vi "ui_Library Two Button Dialog.vi"(1 "F button name (\"Cancel\")":string="Cancel", 2 "T button name (\"OK\")":string="OK", 3 "message":string) -> (0 "T button?":bool)   [LabVIEW 2012]
doc: "Drop-in replacement for LabVIEW's \"Two Button Dialog\" which, at least up to LabVIEW version 7.1, has the nasty property that it blocks the user interface thread while open. The UI thread is required not just for display updates but also for VI loading and instantiation. Thus, using the standard \"Two Button Dialog\" might prevent essential background tasks from doing their job. Since this subVI is implemented in LabVIEW, it does not suffer from this problem. Its connector pane layout is identical so that a simple diagram replace will work."
panel:
  out "message box":string
  in  "F button":bool
  in  "T button":bool
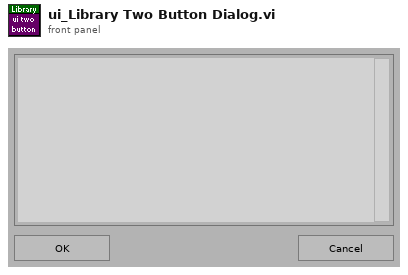
[diagram p1: front panel]
types:
  T1 = typedef "eventvkey.ctl" = enum16{"ASCII", "Enter", "Return", "Shift", "Ctrl", "Alt", "Cmd", "Opt", "Caps", "NumLock", "Clear", "Break", "Up", "Down", "Left", "Right", "Insert", "Delete", "Home", "End", "PageUp", "PageDown", "Escape", "Help", "Pause", "ScrollLock", "F1", "F2", "F3", "F4", "F5", "F6", "F7", "F8", "F9", "F10", "F11", "F12", "F13", "F14", "F15", "F16", "F17", "F18", "F19", "F20", "F21", "F22", "F23", "F24", "Play", "VolumeUp", "VolumeDown", "Mute", "Two Byte Char"}
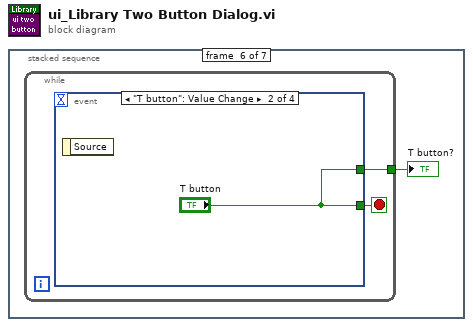
[diagram p0: block diagram]
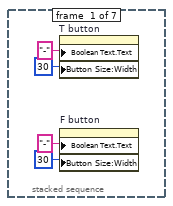
[diagram p2: hidden frame]
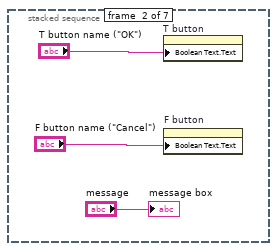
[diagram p3: hidden frame]
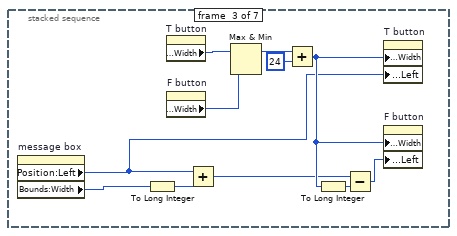
[diagram p4: hidden frame]
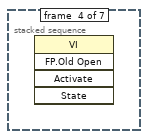
[diagram p5: hidden frame]
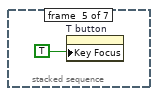
[diagram p6: hidden frame]
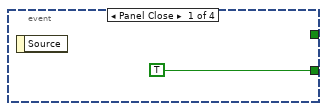
[diagram p7: hidden frame]
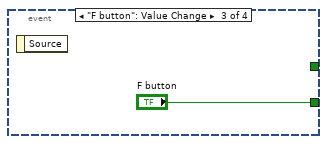
[diagram p8: hidden frame]
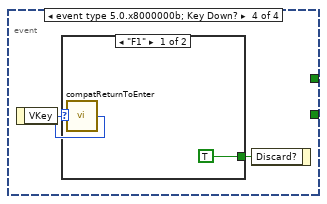
[diagram p9: hidden frame]
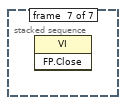
[diagram p11: hidden frame]
diagram:
  n1 = stacked-sequence {
    frame #0 {
      n2 = property on="T button" class="Bool"("Boolean Text.Text"="-", "Button Size:Width"=u32 30) -> ()  [unwired: 2 in, 2 out]
      n3 = property on="F button" class="Bool"("Boolean Text.Text"="-", "Button Size:Width"=u32 30) -> ()  [unwired: 2 in, 2 out]
    }
    frame #1 {
      n4 = property on="T button" class="Bool"("Boolean Text.Text"="T button name (\"OK\")") -> ()  [unwired: 2 in, 2 out]
      n5 = property on="F button" class="Bool"("Boolean Text.Text"="F button name (\"Cancel\")") -> ()  [unwired: 2 in, 2 out]
      "message box" <- "message"
    }
    frame #2 {
      n6 = property on="message box" class="Str"() -> ("Position:Left"=w9:i32, "Bounds:Width"=w8:u32)  [unwired: 2 in, 2 out]
      n7 = To Long Integer(number=w8) -> (32bit integer=w14:i32)
      n8 = property on="T button" class="Bool"() -> ("Button Size:Width"=w18:u32)  [unwired: 2 in, 2 out]
      n9 = property on="F button" class="Bool"() -> ("Button Size:Width"=w17:u32)  [unwired: 2 in, 2 out]
      n10 = Add(x=w9, y=w14) -> (x+y=w12:i32)
      n11 = Max & Min(x=w18, y=w17) -> (max(x,y)=w16:u32)  [unwired: 1 out]
      n12 = Add(x=w16, y=u32 24) -> (x+y=w13:u32)
      n13 = To Long Integer(number=w13) -> (32bit integer=w11:i32)
      n14 = Subtract(x=w12, y=w11) -> (x-y=w10:i32)
      n15 = property on="T button" class="Bool"("Button Size:Width"=w13, "Position:Left"=w9) -> ()  [unwired: 2 in, 2 out]
      n16 = property on="F button" class="Bool"("Button Size:Width"=w13, "Position:Left"=w10) -> ()  [unwired: 2 in, 2 out]
    }
    frame #3 {
      n17 = invoke class="VI" method="FP.Old Open"() -> ()  [unwired: 5 in, 5 out]
    }
    frame #4 {
      n18 = property on="T button" class="Bool"("Key Focus"=TRUE) -> ()  [unwired: 2 in, 2 out]
    }
    frame #5 {
      n19 = while {
        tunnel: [w22] -> w20
        stop <- w21 stop-if-true
        n20 = event shown="[1] \"T button\": Value Change" {
          selector: _ -> [_ _ _ _]
          dyn-events: _ -> [_ _ _ _]
          timeout: _ -> [_ _ _ _]
          tunnel: [_ "T button" _ _] -> w22
          tunnel: [TRUE "T button" "F button" _] -> w21
          event Panel Close {
            n21 = event-data() -> ()  [unwired: 1 in, 1 out]
          }
          event "T button": Value Change {
            n22 = event-data() -> ()  [unwired: 1 in, 1 out]
          }
          event "F button": Value Change {
            n23 = event-data() -> ()  [unwired: 1 in, 1 out]
          }
          event event type 5.0.x8000000b; Key Down? {
            n24 = event-data() -> ("VKey"=w26:T1)  [unwired: 1 in]
            n25 = call <vilib>:"compatReturnToEnter.vi"("VKey"=w26) -> ("VKey"=w28:T1)
            n26 = case shown="\"F1\"" w28 {
              tunnel: [TRUE ("Discard?") _] -> w27
              frame "F1" {
              }
              frame Default {
              }
            }
            n27 = event-data("Discard?"=w27) -> ()  [unwired: 1 in, 1 out]
          }
        }
      }
      "T button?" <- w20
    }
    frame #6 {
      n28 = invoke class="VI" method="FP.Close"() -> ()  [unwired: 3 in, 3 out]
    }
  }
